vi "dvp Vi Get Strobe Driver.vi"(10 "pStrobeDriver":u32(ring) items=["FRAME_DURATION", "TIMER_LOGIC", "SENSOR_STROBE"], 11 "handle":u32) -> (2 "pStrobeDriver out":u32(ring) items=["FRAME_DURATION", "TIMER_LOGIC", "SENSOR_STROBE"], 3 "function return":u32(ring))   [LabVIEW 2018, in "LabViewDVPCamera.lvlib"]
doc: "LabviewDvp2Api dvpStatus dvpViGetStrobeDriver(dvpHandle handle, dvpStrobeDriver *pStrobeDriver);"
uses:
  LabViewDVPCamera.lvlib
  LabViewDVPCamera/LabViewDVPCamera.dll
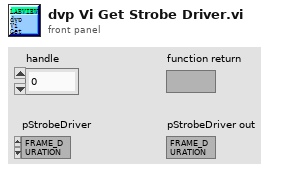
[diagram p1: front panel]
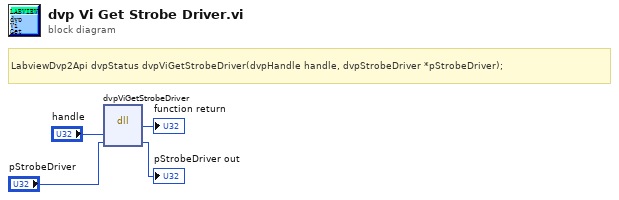
[diagram p0: block diagram]
diagram:
  # "LabviewDvp2Api dvpStatus dvpViGetStrobeDriver(dvpHandle handle, dvpStrobeDriver *pStrobeDriver);"
  n1 = dll-call lib="C:/Program Files (x86)/DVP2 Labview cn 64/Sample/LabViewDVPCamera/LabViewDVPCamera.*" fn="dvpViGetStrobeDriver"("handle"="handle", "pStrobeDriver"="pStrobeDriver") -> (→"function return":u32, "pStrobeDriver"=→"pStrobeDriver out":u32)  [unwired: 4 in, 2 out]
